vi "Panel Reinit.vi"(8 "Error In":errorcluster, 11 "VI Ref":refnum<vi>) -> (0 "Error Out":errorcluster)   [LabVIEW 2019]
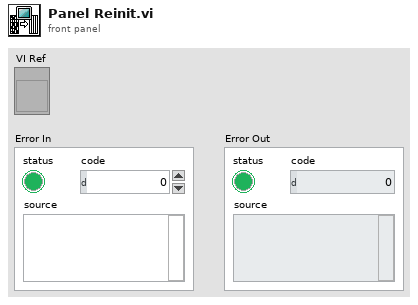
[diagram p1: front panel]
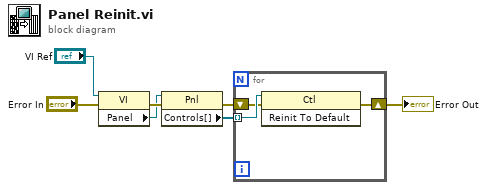
[diagram p0: block diagram]
diagram:
  n1 = property class="VI"(reference="VI Ref", error in="Error In") -> (error out=w5:errorcluster, "Panel"=w2:refnum<vi>)  [unwired: 1 out]
  n2 = property class="Pnl"(reference=w2, error in=w5) -> (error out=w4:errorcluster, "Controls[]"=w3:refnum<vi>[])  [unwired: 1 out]
  n3 = for {
    tunnel: w3 -> [w10] mode=indexing
    shift-right: [w8] -> w7
    shift-left: w4 -> [w9]
    n4 = invoke class="Ctl" method="Reinit To Default"(reference=w10, error in=w9) -> (error out=w8:errorcluster)  [unwired: 1 in, 2 out]
  }
  "Error Out" <- w7
